vi "Seconds to String Times include H_M_S.vi"(11 "Seconds":dbl) -> (3 "concatenated string":string)   [LabVIEW 2021]
panel:
  out "Сʱ":i32
  out "分钟":i32
  out "秒":i32
  out "x-y":dbl
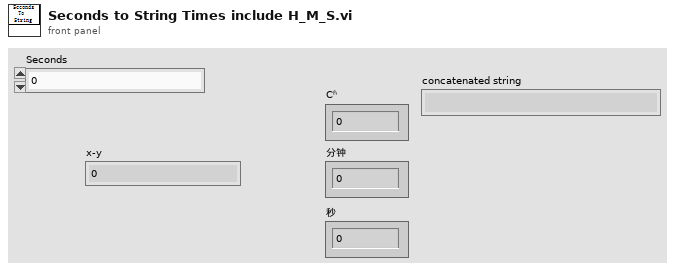
[diagram p1: front panel]
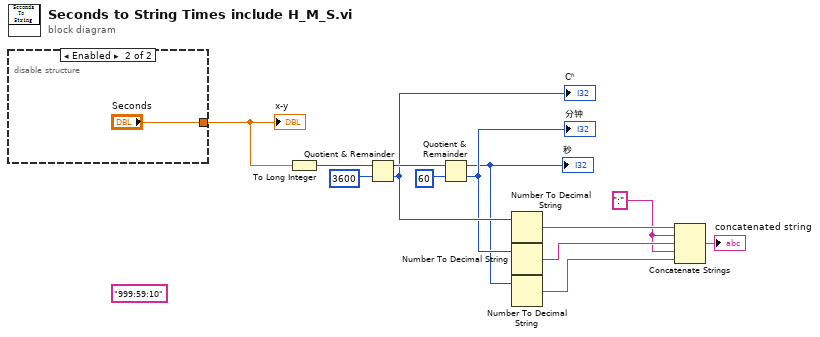
[diagram p0: block diagram]
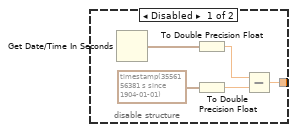
[diagram p2: hidden frame]
diagram:
  w3 = ":" ("string")
  (unwired) "999:59:10" ("RunTime")
  n1 = disable-structure shown="Enabled" {
    disable-tunnel: [w14 "Seconds"] -> w9
    frame Disabled {
      n2 = Get Date/Time In Seconds() -> (seconds since 1Jan1904=w18:timestamp)
      n3 = To Double Precision Float(number=w18) -> (double precision float=w15:dbl)
      n4 = To Double Precision Float(number=timestamp(3556156381.577 s since 1904-01-01) ("current time")) -> (double precision float=w16:dbl)
      n5 = Subtract(x=w15, y=w16) -> (x-y=w14:dbl)
    }
    frame Enabled {
    }
  }
  "x-y" <- w9
  n6 = To Long Integer(number=w9) -> (32bit integer=w13:i32)
  n7 = Quotient & Remainder(x=w13, y=3600) -> (x-y*floor(x/y)=w12:i32, floor(x/y)=w8:i32)
  "Сʱ" <- w8
  n8 = Quotient & Remainder(x=w12, y=60) -> (x-y*floor(x/y)=w6:i32, floor(x/y)=w7:i32)
  "分钟" <- w7
  "秒" <- w6
  n9 = Number To Decimal String(number=w8) -> (decimal integer string=w5:string)  [unwired: 1 in]
  n10 = Number To Decimal String(number=w7) -> (decimal integer string=w4:string)  [unwired: 1 in]
  n11 = Number To Decimal String(number=w6) -> (decimal integer string=w2:string)  [unwired: 1 in]
  n12 = Concatenate Strings(w5, w3, w4, w3, w2) -> (→"concatenated string":string)
